vi "PV HLT5xx mass.vi"(7 "Adress of unit":u16=1 min=1 max=999 step=1, 8 "error in (no error)":errorcluster, 9 "set mass [amu]":u16(ring)=2 items=["mass 2", "mass 3", "mass 4"], 10 "Parameter\nread only<->describe":bool, 11 "VISA session":refnum<visa-resource-name>) -> (0 "error out":errorcluster, 1 "mass [amu] out":u16(ring)=2 items=["mass 2", "mass 3", "mass 4"], 2 "response (data)":string, 3 "dup VISA session":refnum<visa-resource-name>)   [LabVIEW 2021, in "Pfeiffer Vacuum.lvlib"]
doc: "This VI allows you to set or check the \"Mass [amu] (Para 642)\" on the SmartTest (HLT5xx)."
uses:
  <instrlib>/Pfeiffer Vacuum/Pfeiffer Vacuum.lvlib
panel:
  # "Mass [amu]"
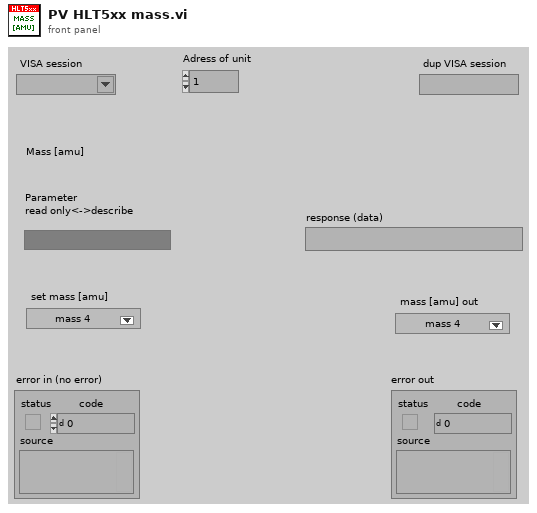
[diagram p1: front panel]
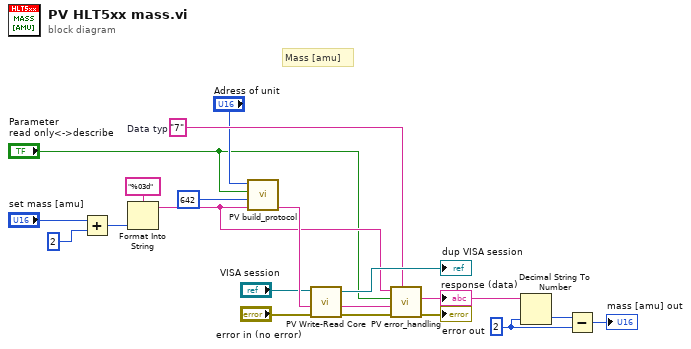
[diagram p0: block diagram]
diagram:
  w1 = u16 2
  w14 = "7"  # Data typ
  # "Mass [amu]"
  n1 = Add(x="set mass [amu]", y=u16 2) -> (x+y=w6:u16)
  n2 = Format Into String(format string="%03d" ("Format-String"), w6) -> (resulting string=w15:string)  [unwired: 2 in, 1 out]
  n3 = call <instrlib>:"PV build_protocol.vi"("Data"=w15, "Parameter-number"=u16 642, "parameter\nread<->describe"="Parameter\nread only<->describe", "Adress"="Adress of unit") -> ("output"=w19:string)  [unwired: 3 in]
  n4 = call <instrlib>:"PV Write-Read Core.vi"("error in"="error in (no error)", "Write data in"=w19, "VISA session"="VISA session") -> ("error out"=w17:errorcluster, "response (data) out"=w18:string, "dup VISA session"=→"dup VISA session":refnum<visa-resource-name>)  [unwired: 2 in]
  n5 = call <instrlib>:"PV error_handling.vi"("Data Typ in"=w14, "error in"=w17, "response (data) in"=w18, "Parameter\nread only<->describe"="Parameter\nread only<->describe", "data in"=w15) -> ("error out"=→"error out":errorcluster, "Data out"=w12:string)  [unwired: 4 in, 1 out]
  "response (data)" <- w12
  n6 = Decimal String To Number(string=w12, default (0L)=w1) -> (number=w3:u16)  [unwired: 1 in, 1 out]
  n7 = Subtract(x=w3, y=w1) -> (x-y=→"mass [amu] out":u16)
